vi "ryerror_obtain.vi"(8 "error in (no error)":errorcluster) -> (0 "error out":errorcluster, 1 "error queue":refnum<queue>)   [LabVIEW 2017]
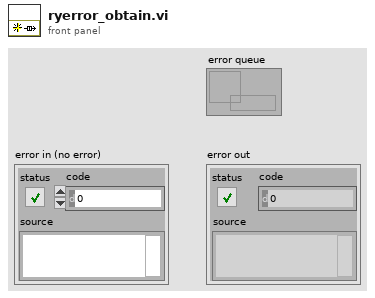
[diagram p1: front panel]
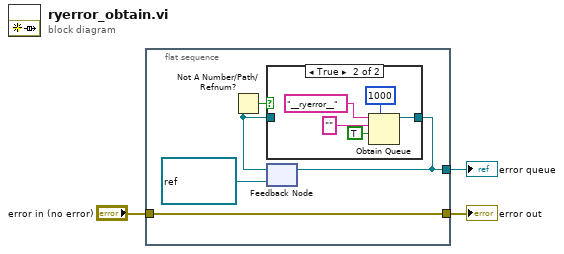
[diagram p0: block diagram]
diagram:
  n1 = flat-sequence {
    tunnel: [w8] -> w1
    tunnel: [w5] -> w3
    tunnel: "error in (no error)" -> [w5]
    frame #0 {
      n2 = feedback #1(refnum<queue> refnum ("queue out")) -> (w7:refnum<queue>)
      n3 = Not A Number/Path/Refnum?(number/path/refnum=w7) -> (NaN/Path/Refnum?=w6:bool)
      n4 = case shown="True" w6 {
        tunnel: [w9 w12] -> w8
        tunnel: w7 -> [w9 _]
        frame False {
        }
        frame True {
          n5 = Obtain Queue(max queue size (-1, unlimited)=1000, name (unnamed)="__ryerror__", element data type="", create if not found? (T)=TRUE) -> (queue out=w12:refnum<queue>)  [unwired: 1 in, 2 out]
        }
      }
      n6 = feedback-in #1(w8) -> ()
    }
  }
  "error out" <- w3
  "error queue" <- w1
